vi "in_2d interp.vi"(6 "yi":dbl[][](array[numeric]), 7 "method":i32(ring) items=["nearest", "bilinear", "bicubic", "bicubic spline"], 8 "xi":dbl[][](array[numeric]), 9 "Y":dbl[](array[numeric]), 10 "X":dbl[](array[numeric]), 11 "Z":dbl[][](array[numeric])) -> (3 "zi":dbl[][](array[numeric]))   [LabVIEW 2017, in "NI_Gmath.lvlib"]
uses:
  NI_Gmath.lvlib
  A x Vector.vi
  Real Dot Product.vi
  NI_AALBase.lvlib
  NI_AALPro.lvlib
panel:
  # "Interpolate 2D"
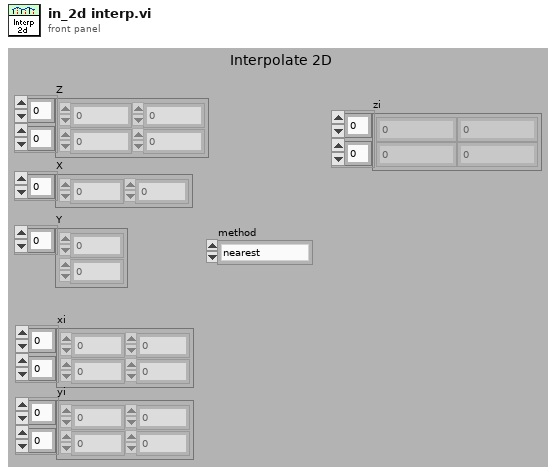
[diagram p1: front panel]
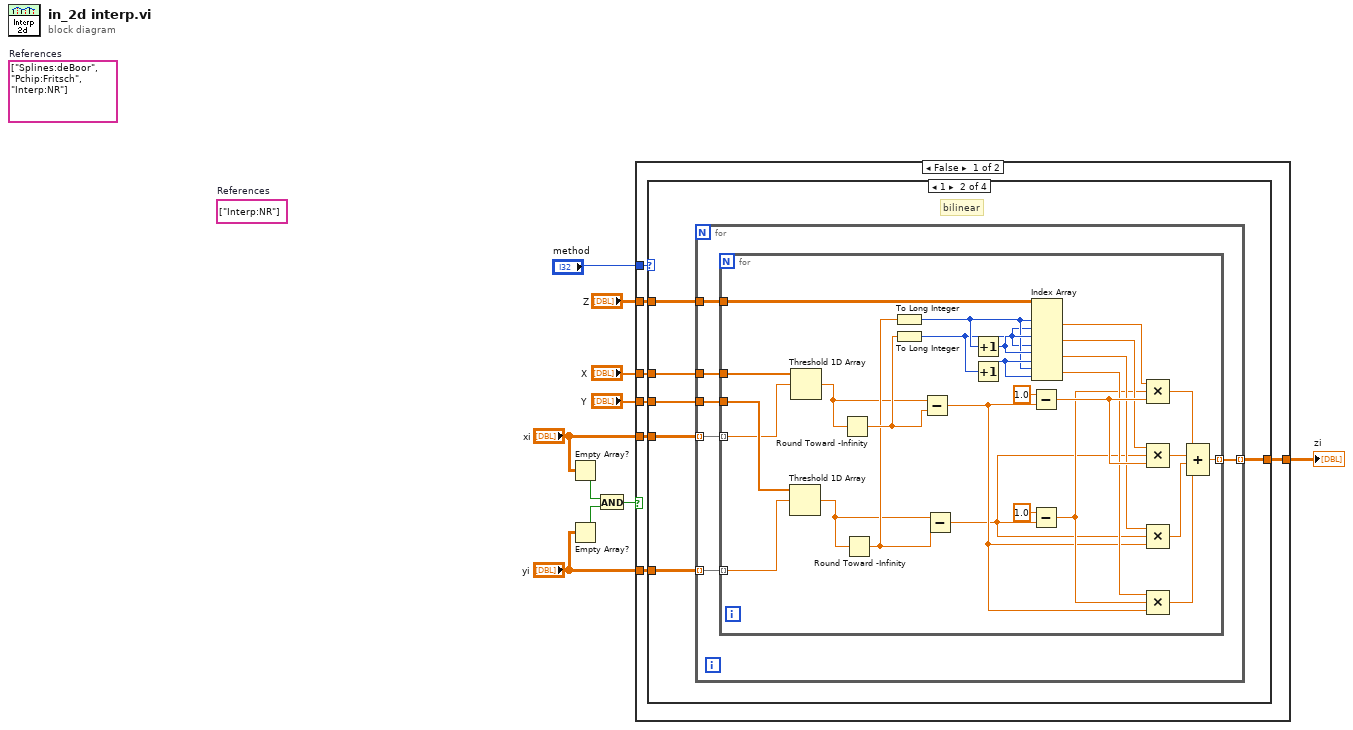
[diagram p0: block diagram]
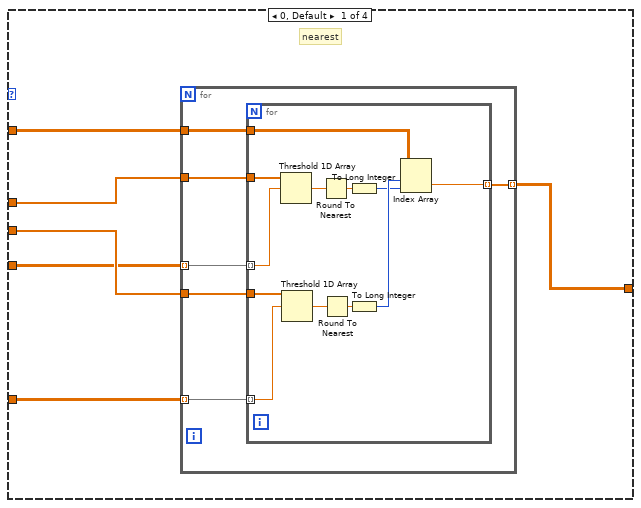
[diagram p2: hidden frame]
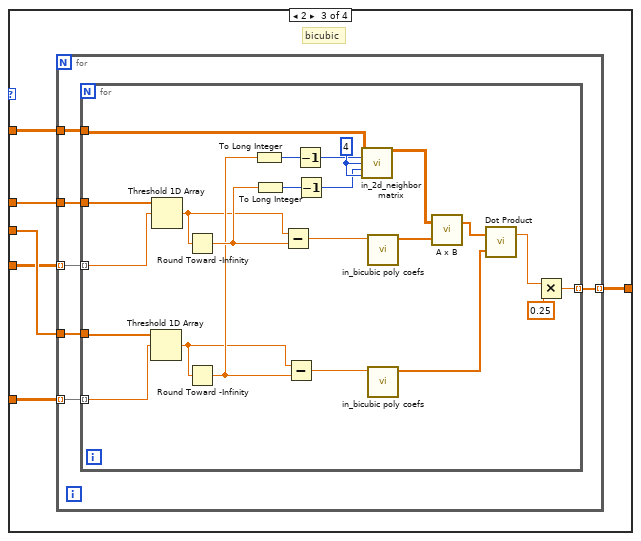
[diagram p3: hidden frame]
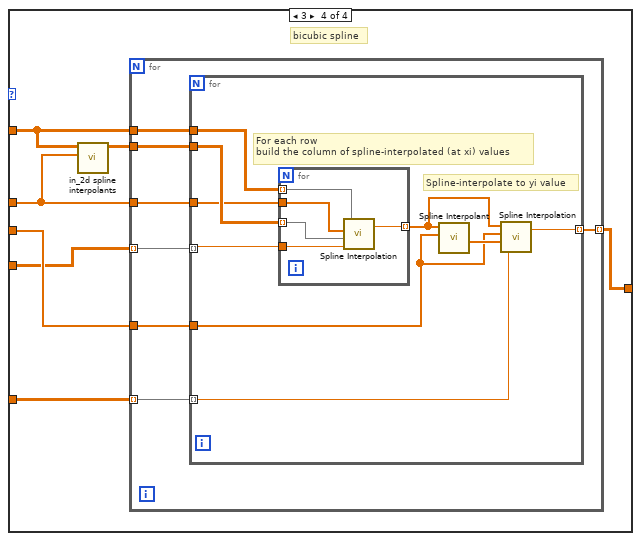
[diagram p4: hidden frame]
diagram:
  (unwired) string[] ["Interp:NR"]  # References
  (unwired) string[] ["Splines:deBoor", "Pchip:Fritsch", "Interp:NR"]  # References
  n1 = Empty Array?(array="xi") -> (empty?=w2:bool)
  n2 = Empty Array?(array="yi") -> (empty?=w3:bool)
  n3 = And(x=w2, y=w3) -> (x .and. y?=w1:bool)
  n4 = case shown="False" w1 {
    tunnel: "method" -> [w17 _]
    tunnel: "X" -> [w16 _]
    tunnel: "Y" -> [w15 _]
    tunnel: "Z" -> [w14 w145]
    tunnel: [w13 w145] -> w6
    tunnel: "xi" -> [w12 _]
    tunnel: "yi" -> [w11 _]
    frame False {
      n5 = case shown="1" w17 {
        tunnel: w11 -> [w23 w43 w83 w123]
        tunnel: w15 -> [w22 w47 w87 w120]
        tunnel: w16 -> [w21 w46 w86 w118]
        tunnel: w14 -> [w20 w45 w85 w119]
        tunnel: [w19 w42 w82 w121] -> w13
        tunnel: w12 -> [w18 w44 w84 w117]
        frame 0, Default {
          # "nearest"
          n6 = for {
            tunnel: w22 -> [w25]
            tunnel: w23 -> [w24] mode=indexing
            tunnel: w21 -> [w29]
            tunnel: w20 -> [w28]
            tunnel: [w27] -> w19 mode=indexing
            tunnel: w18 -> [w26] mode=indexing
            n7 = for {
              tunnel: w29 -> [w40]
              tunnel: w28 -> [w39]
              tunnel: [w37] -> w27 mode=indexing
              tunnel: w26 -> [w32] mode=indexing
              tunnel: w25 -> [w35]
              tunnel: w24 -> [w33] mode=indexing
              n8 = Threshold 1D Array(2:w32, 3:w40) -> (0:w41:dbl)  [unwired: 1 in]
              n9 = Threshold 1D Array(2:w33, 3:w35) -> (0:w36:dbl)  [unwired: 1 in]
              n10 = Round To Nearest(number=w41) -> (nearest integer value=w38:dbl)
              n11 = Round To Nearest(number=w36) -> (nearest integer value=w34:dbl)
              n12 = To Long Integer(number=w38) -> (32bit integer=w30:i32)
              n13 = To Long Integer(number=w34) -> (32bit integer=w31:i32)
              n14 = Index Array(array=w39, index (row)=w31, index (col)=w30) -> (element=w37:dbl)
            }
          }
        }
        frame 1 {
          # "bilinear"
          n15 = for {
            tunnel: w47 -> [w53]
            tunnel: w46 -> [w52]
            tunnel: w45 -> [w51]
            tunnel: w44 -> [w50] mode=indexing
            tunnel: w43 -> [w49] mode=indexing
            tunnel: [w48] -> w42 mode=indexing
            n16 = for {
              tunnel: w53 -> [w81]
              tunnel: w49 -> [w67] mode=indexing
              tunnel: w52 -> [w63]
              tunnel: w51 -> [w80]
              tunnel: w50 -> [w62] mode=indexing
              tunnel: [w68] -> w48 mode=indexing
              n17 = Threshold 1D Array(2:w67, 3:w81) -> (0:w55:dbl)  [unwired: 1 in]
              n18 = Threshold 1D Array(2:w62, 3:w63) -> (0:w54:dbl)  [unwired: 1 in]
              n19 = Round Toward -Infinity(1:w54) -> (0:w59:dbl)
              n20 = Round Toward -Infinity(1:w55) -> (0:w57:dbl)
              n21 = To Long Integer(number=w57) -> (32bit integer=w65:i32)
              n22 = To Long Integer(number=w59) -> (32bit integer=w64:i32)
              n23 = Subtract(x=w54, y=w59) -> (x-y=w58:dbl)
              n24 = Subtract(x=w55, y=w57) -> (x-y=w56:dbl)
              n25 = Increment(x=w65) -> (x+1=w79:i32)
              n26 = Increment(x=w64) -> (x+1=w78:i32)
              n27 = Subtract(x=1.0, y=w58) -> (x-y=w74:dbl)
              n28 = Subtract(x=1.0, y=w56) -> (x-y=w60:dbl)
              n29 = Index Array(array=w80, index (row) #1=w65, index (col) #1=w64, index (row) #2=w79, index (col) #2=w64, index (row) #3=w79, index (col) #3=w78, index (row) #4=w65, index (col) #4=w78) -> (element #1=w75:dbl, element #2=w61:dbl, element #3=w73:dbl, element #4=w72:dbl)
              n30 = Compound Arithmetic op=MULTIPLY(w75, w60, w74) -> (w71:dbl)
              n31 = Compound Arithmetic op=MULTIPLY(w61, w56, w74) -> (w70:dbl)
              n32 = Compound Arithmetic op=MULTIPLY(w73, w56, w58) -> (w66:dbl)
              n33 = Compound Arithmetic op=MULTIPLY(w72, w60, w58) -> (w69:dbl)
              n34 = Compound Arithmetic op=ADD(w71, w70, w66, w69) -> (w68:dbl)
            }
          }
        }
        frame 2 {
          # "bicubic"
          n35 = for {
            tunnel: w87 -> [w93]
            tunnel: w86 -> [w92]
            tunnel: w85 -> [w91]
            tunnel: w84 -> [w90] mode=indexing
            tunnel: w83 -> [w89] mode=indexing
            tunnel: [w88] -> w82 mode=indexing
            n36 = for {
              tunnel: w93 -> [w116]
              tunnel: w89 -> [w104] mode=indexing
              tunnel: w92 -> [w115]
              tunnel: w91 -> [w113]
              tunnel: w90 -> [w105] mode=indexing
              tunnel: [w107] -> w88 mode=indexing
              w112 = 4 ("row length")
              n37 = Threshold 1D Array(2:w104, 3:w116) -> (0:w95:dbl)  [unwired: 1 in]
              n38 = Threshold 1D Array(2:w105, 3:w115) -> (0:w94:dbl)  [unwired: 1 in]
              n39 = Round Toward -Infinity(1:w94) -> (0:w99:dbl)
              n40 = Round Toward -Infinity(1:w95) -> (0:w97:dbl)
              n41 = To Long Integer(number=w97) -> (32bit integer=w114:i32)
              n42 = To Long Integer(number=w99) -> (32bit integer=w111:i32)
              n43 = Subtract(x=w94, y=w99) -> (x-y=w98:dbl)
              n44 = Subtract(x=w95, y=w97) -> (x-y=w96:dbl)
              n45 = Decrement(x=w114) -> (x-1=w110:i32)
              n46 = Decrement(x=w111) -> (x-1=w109:i32)
              n47 = call "in_2d_neighbor matrix.vi"("array"=w113, "row index"=w110, "row length"=w112, "col index"=w109, "col length"=w112) -> ("subarray"=w103:dbl[][])  [unwired: 10 in]
              n48 = call "in_bicubic poly coefs.vi"("t"=w98) -> ("bicubic polynomial"=w100:dbl[])  [unwired: 10 in]
              n49 = call "in_bicubic poly coefs.vi"("t"=w96) -> ("bicubic polynomial"=w101:dbl[])  [unwired: 10 in]
              n50 = call-poly "A x B.vi"("Vector"=w100, "A"=w103) -> ("A x Vector"=w102:dbl[])  [unwired: 1 out]
              n51 = call-poly "Dot Product.vi"("Y Vector"=w101, "X Vector"=w102) -> ("X * Y"=w108:dbl)  [unwired: 1 out]
              n52 = Multiply(x=w108, y=0.25) -> (x*y=w107:dbl)
            }
          }
        }
        frame 3 {
          # "bicubic spline"
          n53 = call "in_2d spline interpolants.vi"("X row"=w118, "Z matrix"=w119) -> ("2d spline interpolants"=w122:dbl[][])  [unwired: 9 in]
          n54 = for {
            tunnel: w120 -> [w130]
            tunnel: w119 -> [w125]
            tunnel: w123 -> [w129] mode=indexing
            tunnel: w122 -> [w127]
            tunnel: w117 -> [w128] mode=indexing
            tunnel: w118 -> [w126]
            tunnel: [w124] -> w121 mode=indexing
            n55 = for {
              tunnel: w130 -> [w132]
              tunnel: w129 -> [w131] mode=indexing
              tunnel: w128 -> [w133] mode=indexing
              tunnel: w127 -> [w139]
              tunnel: w126 -> [w134]
              tunnel: w125 -> [w138]
              tunnel: [w135] -> w124 mode=indexing
              # "Spline-interpolate to yi value"
              # "For each row\nbuild the column of spline-interpolated (at xi) values"
              n56 = for {
                tunnel: w139 -> [w144] mode=indexing
                tunnel: w138 -> [w143] mode=indexing
                tunnel: [w142] -> w136 mode=indexing
                tunnel: w134 -> [w141]
                tunnel: w133 -> [w140]
                n57 = call "Spline Interpolation.vi"("x value"=w140, "Interpolant"=w144, "X"=w141, "Y"=w143) -> ("interpolation value"=w142:dbl)  [unwired: 1 out]
              }
              n58 = call "Spline Interpolant.vi"("X"=w132, "Y"=w136) -> ("Interpolant"=w137:dbl[])  [unwired: 2 in, 1 out]
              n59 = call "Spline Interpolation.vi"("x value"=w131, "Interpolant"=w137, "X"=w132, "Y"=w136) -> ("interpolation value"=w135:dbl)  [unwired: 1 out]
            }
          }
        }
      }
    }
    frame True {
    }
  }
  "zi" <- w6
